vi "dust_list.vi"() -> ()   [LabVIEW 2013]
uses:
  Private/Controls/Dust_list.ctl
panel:
  out "Array":T1[](array[typedef])
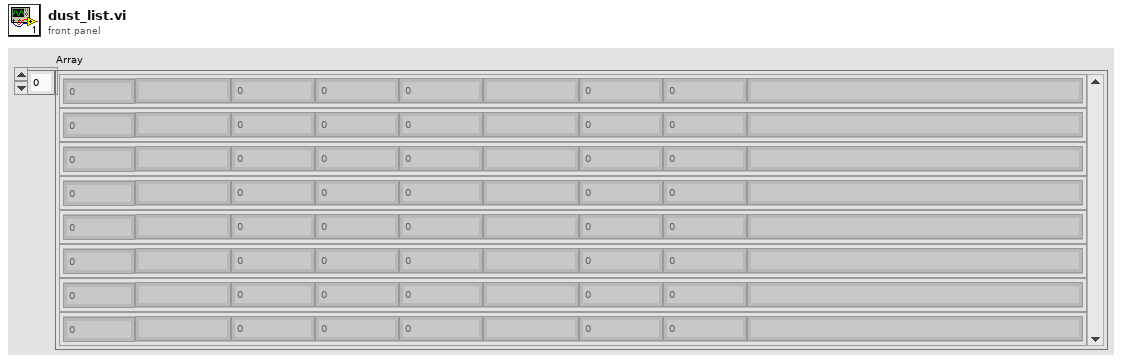
[diagram p1: front panel]
types:
  T1 = typedef "Dust_list.ctl" = cluster{"id_dust_type":dbl, "dust_name":string, "batch_number":dbl, "dust_density":dbl, "source_weight":dbl, "size":string, "bottle_weight":dbl, "dust_weight":dbl, "comments":string}
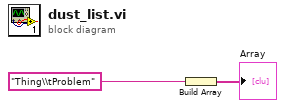
[diagram p0: block diagram]
diagram:
  n1 = Build Array("Thing\\tProblem") -> (→"Array":string[])
